vi "Get Task Performance.vi"(4 "Error In":errorcluster, 6 "Performance Counters":T1(ring)=enum."% Processor Time", 7 "Instance Name":string="LabVIEW") -> (0 "Error Out":errorcluster, 3 "Counter Value":dbl)   [LabVIEW 2014, in "Managing Executables.lvlib"]
uses:
  Managing Executables.lvlib
  Timing/Timing.lvlib
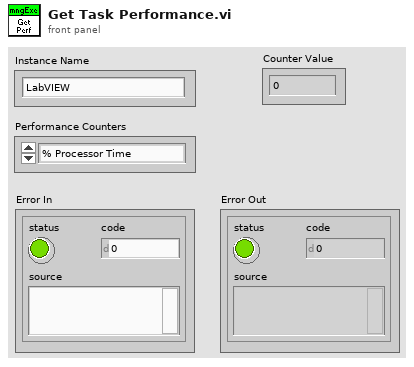
[diagram p1: front panel]
types:
  T1 = enum16{"% Privileged Time", "% Processor Time", "% User Time", "Creating Process ID", "Elapsed Time", "Handle Count", "ID Process", "IO Data Bytes/sec", "IO Data Operations/sec", "IO Other Bytes/sec", "IO Other Operations/sec", "IO Read Bytes/sec", "IO Read Operations/sec", "IO Write Bytes/sec", "IO Write Operations/sec", "Page Faults/sec", "Page File Bytes", "Page File Bytes Peak", "Pool Nonpaged Bytes", "Pool Paged Bytes", "Priority Base", "Private Bytes", "Thread Count", "Virtual Bytes", "Virtual Bytes Peak", "Working Set", "Working Set - Private", "Working Set Peak"}
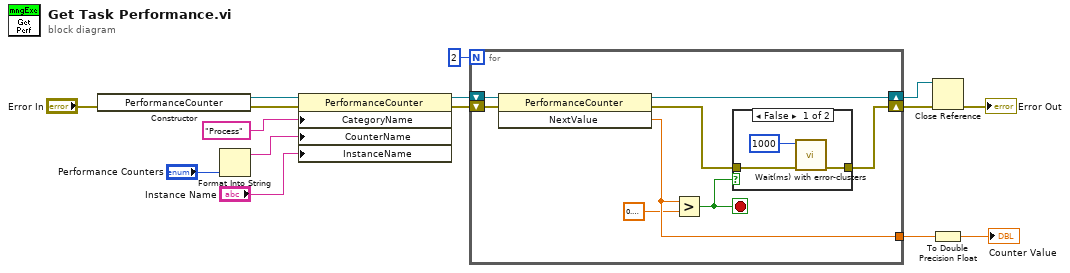
[diagram p0: block diagram]
diagram:
  n1 = constructor class="PerformanceCounter"(error in="Error In") -> (reference out=w9:refnum<k24>, error out=w3:errorcluster)  [unwired: 2 in, 1 out]
  n2 = Format Into String("Performance Counters") -> (resulting string=w6:string)  [unwired: 3 in, 1 out]
  n3 = property class="PerformanceCounter"(reference=w9, error in=w3, "CategoryName"="Process" ("Category List 2"), "CounterName"=w6, "InstanceName"="Instance Name") -> (reference out=w8:refnum<k24>, error out=w4:errorcluster)
  n4 = for {
    N: 2 -> [_]
    tunnel: [w20] -> w14
    shift-right: [w23] -> w15
    shift-left: w8 -> [w22]
    shift-right: [w17] -> w12
    shift-left: w4 -> [w21]
    stop <- w16 stop-if-true
    n5 = invoke class="PerformanceCounter" method="NextValue"(reference=w22, error in=w21) -> (reference out=w23:refnum<k24>, error out=w18:errorcluster, "NextValue"=w20:sgl)  [unwired: 1 in]
    n6 = Greater?(x=w20, y=sgl 0.1) -> (0:w16:bool)
    n7 = case shown="False" w16 {
      tunnel: w18 -> [w25 w27]
      tunnel: [w24 w27] -> w17
      frame False {
        n8 = call "Wait(ms) with error-clusters.vi"("Error In"=w25, "wait (msec)"=u32 1000) -> ("Error Out"=w24:errorcluster)  [unwired: 5 in]
      }
      frame True {
      }
    }
  }
  n9 = Close Reference(reference=w15, error in (no error)=w12) -> (error out=→"Error Out":errorcluster)
  n10 = To Double Precision Float(number=w14) -> (double precision float=→"Counter Value":dbl)
